vi "CRC16_Calc.vi"(9 "buffer":u8[](array[numeric]) format="%.0x", 10 "crc":u16) -> (2 "crc 2":u16)   [LabVIEW 2017]
panel:
  in  "len":u32
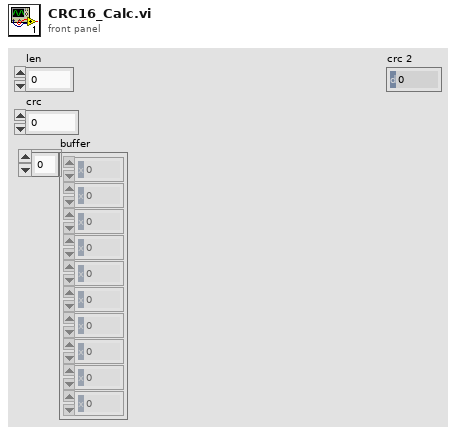
[diagram p1: front panel]
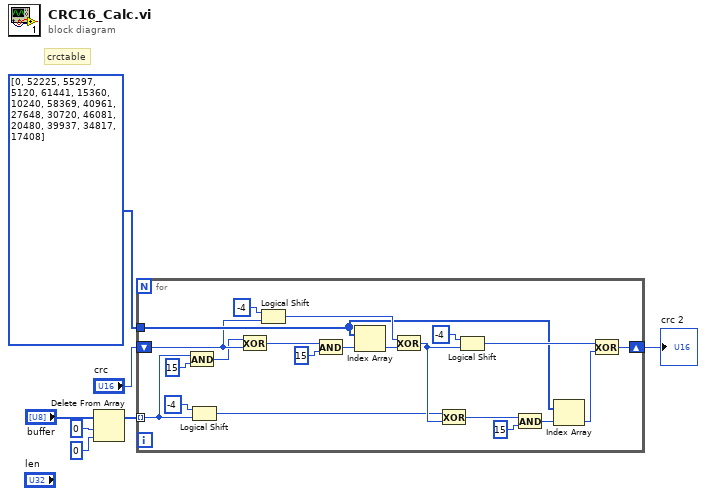
[diagram p0: block diagram]
diagram:
  # "crctable"
  n1 = Delete From Array(array="buffer", length=0, index=0) -> (array with subset deleted=w3:u8[])  [unwired: 1 out]
  n2 = for {
    tunnel: w3 -> [w9] mode=indexing
    tunnel: i32[] [0, 52225, 55297, 5120, 61441, 15360, 10240, 58369, 40961, 27648, 30720, 46081, 20480, 39937, 34817, 17408] -> [w22]
    shift-right: [w21] -> w1
    shift-left: "crc" -> [w20]
    n3 = And(x=w9, y=u8 15) -> (x .and. y?=w8:u8)
    n4 = Logical Shift(y=i16 -4, x=w9) -> (x << y=w11:u8)
    n5 = Exclusive Or(1:w20, 2:w8) -> (0:w16:i32)
    n6 = Logical Shift(y=i16 -4, x=w20) -> (x << y=w27:i32)
    n7 = And(x=w16, y=u16 15) -> (x .and. y?=w17:i32)
    n8 = Index Array(array=w22, index=w17) -> (element=w26:i32)
    n9 = Exclusive Or(1:w26, 2:w27) -> (0:w19:i32)
    n10 = Exclusive Or(1:w19, 2:w11) -> (0:w13:i32)
    n11 = Logical Shift(y=i16 -4, x=w19) -> (x << y=w24:i32)
    n12 = And(x=w13, y=u16 15) -> (x .and. y?=w14:i32)
    n13 = Index Array(array=w22, index=w14) -> (element=w25:i32)
    n14 = Exclusive Or(1:w25, 2:w24) -> (0:w21:i32)
  }
  "crc 2" <- w1
